vi "Send Find Measurements on Disk Message.vi"(8 "error in (no error)":errorcluster, 10 "Measurement Locations":path[](array[path]), 11 "Message Enqueuer in":refnum<class "Message Enqueuer.lvclass">) -> (0 "error out":errorcluster, 3 "Message Enqueuer out":refnum<class "Message Enqueuer.lvclass">)   [LabVIEW 2015, in "Controller Actor.lvlib" / "Find Measurements On Disk Message.lvclass"]
uses:
  Find Measurements On Disk Message.lvclass
  <vilib>/ActorFramework/Message Enqueuer/Message Enqueuer.lvclass
  <vilib>/ActorFramework/Message Enqueuer/Message Enqueuer.lvclass/Message Enqueuer.ctl
  <vilib>/ActorFramework/Message Priority Queue/Priority Enqueue.vi
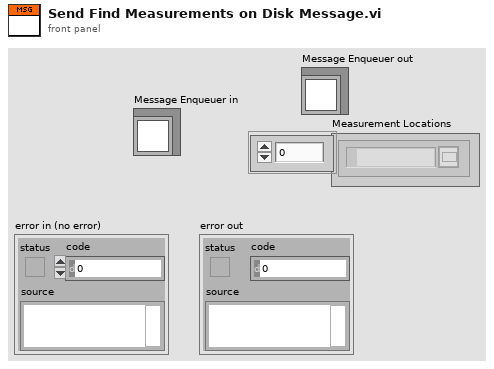
[diagram p1: front panel]
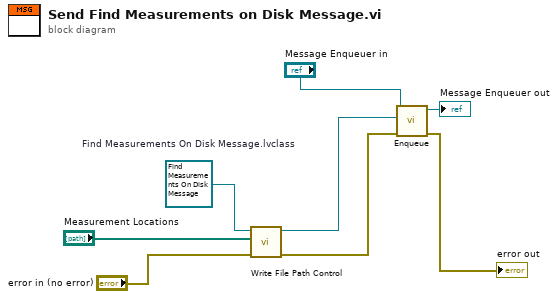
[diagram p0: block diagram]
diagram:
  w8 = refnum<class "Find Measurements On Disk Message.lvclass"> refnum  # Find Measurements On Disk Message.lvclass
  n1 = call "Write File Path Control.vi"("error in (no error)"="error in (no error)", "Measurement Locations"="Measurement Locations", "Load Measurements Message in"=w8) -> ("error out"=w5:errorcluster, "Load Measurements Message out"=w6:refnum<class "Find Measurements On Disk Message.lvclass">)  [unwired: 7 in]
  n2 = call <vilib>:"Enqueue.vi"("error in (no error)"=w5, "Message"=w6, "Message Enqueuer in"="Message Enqueuer in") -> ("error out"=→"error out":errorcluster, "Message Enqueuer out"=→"Message Enqueuer out":refnum<class "Message Enqueuer.lvclass">)  [unwired: 7 in]
